vi "Friction Model(deferred).vi"(5 "cou_f":dbl=2.0 format="%#_13g", 6 "threshold":dbl=0.5 format="%#_13g", 7 "vis_f":dbl format="%#_13g", 10 "RPM":i32[](array[knob]) scale=-200.0..200.0) -> (1 "Voltage":dbl[](array[knob]) scale=-10.0..10.0)   [LabVIEW 2021]
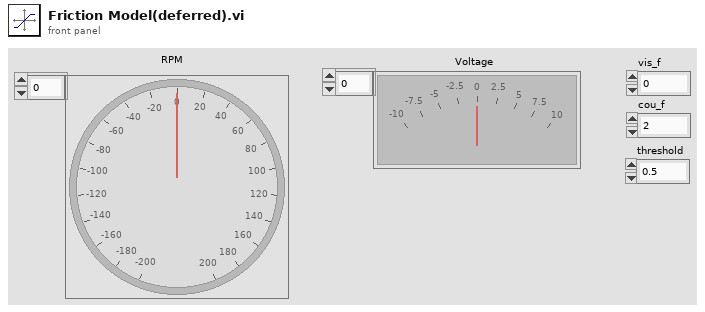
[diagram p1: front panel]
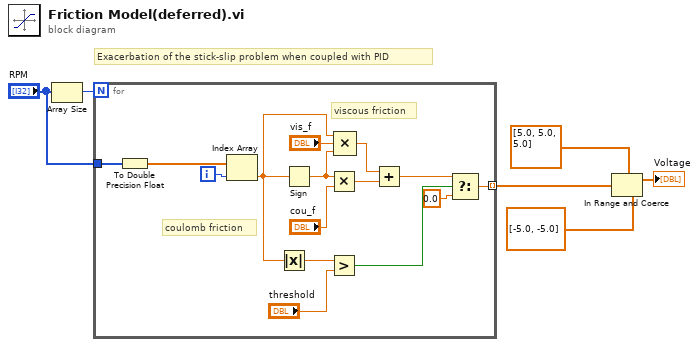
[diagram p0: block diagram]
diagram:
  # "Exacerbation of the stick-slip problem when coupled with PID"
  n1 = Array Size(array="RPM") -> (size(s)=w3:i32)
  n2 = for {
    N: w3 -> [_]
    tunnel: "RPM" -> [w8]
    tunnel: [w15] -> w1 mode=indexing
    i -> [w21]
    # "coulomb friction"
    # "viscous friction"
    n3 = To Double Precision Float(number=w8) -> (double precision float=w7:dbl[])
    n4 = Index Array(array=w7, index=w21) -> (element=w11:dbl)
    n5 = Absolute Value(x=w11) -> (abs(x)=w20:dbl)
    n6 = Sign(1:w11) -> (0:w9:dbl)
    n7 = Multiply(x=w9, y="cou_f") -> (x*y=w13:dbl)
    n8 = Greater?(x=w20, y="threshold") -> (0:w18:bool)
    n9 = Compound Arithmetic op=MULTIPLY(w11, "vis_f", w9) -> (w12:dbl)
    n10 = Add(x=w12, y=w13) -> (x+y=w16:dbl)
    n11 = Select(t=w16, s=w18, f=0.0) -> (s? t:f=w15:dbl)
  }
  n12 = In Range and Coerce(upper limit=dbl[] [5.0, 5.0, 5.0], x=w1, lower limit=dbl[] [-5.0, -5.0]) -> (coerced(x)=→"Voltage":dbl[])  [unwired: 1 out]
